vi "PockelsControl.vi"(8 "Error In":errorcluster, 10 "Laser Power (%)":dbl max=100.0 step=1.0) -> (0 "Error Out":errorcluster)   [LabVIEW 2013]
uses:
  Peripherals Control/Shutter/Typedefs/Shutter state.ctl
  Typedefs/HW config states enum.ctl
  <vilib>/DAQmx/write.llb/DAQmx Write (Analog DBL 1Chan 1Samp).vi
  Global Variables/General Globals.vi
  Global Variables/gl_UI Ctrl Refs.vi
  Peripherals Control/Pockels/Globals/gl_Pockels control globals.vi
  <vilib>/DAQmx/create/channels.llb/DAQmx Create Channel (AO-Voltage-Basic).vi
  <vilib>/DAQmx/miscellaneous.llb/DAQmx Fill In Error Info.vi
panel:
  out "DAQmx Physical Channel":tag="PXI1Slot4/ao0"
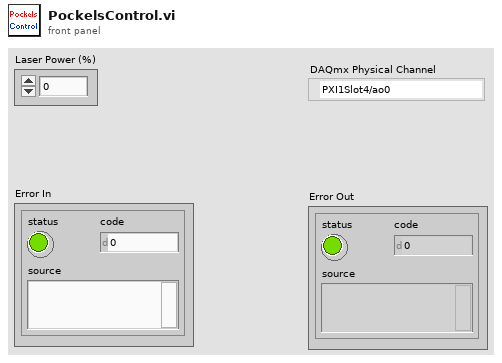
[diagram p1: front panel]
types:
  T1 = typedef "Shutter state.ctl" = enum16{"Closed/Disabled", "Open/Enabled"}
  T2 = typedef "HW config states enum.ctl" = enum16{"Load from file", "Save to file", "Write all", "Read all", "Write XY stage settings", "Write DAQ FPGA settings", "Write Control FPGA settings", "Write Phys Channels", "Clear", "Compare from file"}
  T3 = typedef "Sys Configuration.ctl" = cluster{"XY Stage":T4, "DAQ FPGA":T5, "Control system":T9, "Encoder":T10, "DAQmx Chan":T11, "Computer MAC address":string, "Cam VidRec":T12, "Externalise Triggers":bool, "Laser wavelength (nm)":dbl}
  T4 = typedef "XY Stage config cluster.ctl" = cluster{"COM port":refnum<visa-resource-name>, "XY stage available":bool}
  T5 = typedef "DAQ FPGA config cluster.ctl" = cluster{"Ref":T6, "Target":T7, "Clock Freq (MHz) ":dbl, "input card type":T8, "Samples Wait after Trigger":u16, "AOD fill":u16, "StartupDelay":i32, "Slip Cycle (clock cycles)":u32, "Add Cycle":bool}
  T6 = typedef "FPGA Ref.ctl" = refnum<k20>
  T7 = typedef "nirio_resource_hc.ctl" = tag
  T8 = typedef "FPGA input type AC-DC.ctl" = enum16{"AC Card", "DC Card"}
  T9 = typedef "CTRL system config cluster.ctl" = cluster{"Ethernet opened":bool, "Ethernet Port":u32, "Ctrl FPGA available":bool, "Ctrl FPGA Clock (MHz)":dbl, "Ctrl system MAC address":string, "Control system.Network adapter name":string, "AOD 1 Amplitude":i16, "AOD 2 Amplitude":i16, "AOD 3 Amplitude":i16, "AOD 4 Amplitude":i16, "Data Time Interval (ns)":dbl, "T0 (ns)":dbl, "Ta (ns)":dbl}
  T10 = typedef "Encoder config cluster.ctl" = cluster{"IP address":string, "Port":u16, "Encoder available":bool, "Wheel radius (cm)":dbl}
  T11 = typedef "DAQmx physical channels cluster.ctl" = cluster{"Pockels AO":tag, "Hard shutter AO":tag, "PMT AOs":tag, "Power meter AI":tag}
  T12 = typedef "Cam VidRec HW config setup cluster.ctl" = cluster{"DO flag-Video record":tag, "DO flag-Trial start":tag, "VidRec available":bool}
  T13 = typedef "UI ctrl refs cluster.ctl" = cluster{"Top level VI path":path, "Top level VI ref":refnum<vi>, "User menu ref":refnum<k9>, "Sub Panel control":refnum<vi>, "Imaging Param Tab":refnum<vi>, "Occurrence-Start drivers":refnum<k4>, "Occurrence-Speed logging initialised":refnum<k4>, "Occurrence-XYZ stage initialised":refnum<k4>, "Exit button":refnum<vi>, "Status ind":refnum<vi>, "Return to Origin":refnum<vi>, "Speed Logging":refnum<vi>, "Time Lapse":refnum<vi>, "Live Imaging":refnum<vi>, "AOL Z Stack":refnum<vi>, "Motor Z Stack":refnum<vi>, "Funct Acq button":refnum<vi>, "Hard Shutter":refnum<vi>, "Virtual Shutter":refnum<vi>, "Laser Power":refnum<vi>, "AOL Mode":refnum<vi>, "Frame Size":refnum<vi>, "Field of View":refnum<vi>, "Dwell Time":refnum<vi>, "Zoom":refnum<vi>, "AOL Z":refnum<vi>, "Objective":refnum<vi>, "Axis":refnum<vi>, "Paths & Names":refnum<vi>, "Experiment folder path (ind.)":refnum<vi>, "Last State (Ind.)":refnum<vi>, "Laser wavelength ind (nm)":refnum<vi>, "Averages":refnum<vi>, "Angle (degrees)":refnum<vi>, "X centre":refnum<vi>, "Y centre":refnum<vi>, "Plane Mode":refnum<vi>, "# Planes":refnum<vi>, "Z Start":refnum<vi>, "Z Stop":refnum<vi>, "Z Step":refnum<vi>, "PMT 1":refnum<vi>, "PMT 2":refnum<vi>, "Stage XYZ Position":refnum<vi>, "Pockels@Z Start":refnum<vi>, "Pockels@Z Stop":refnum<vi>, "Obtain Z Start":refnum<vi>, "Obtain Z Stop":refnum<vi>, "Live stim.trig.period":refnum<vi>, "Live stim.trig.enable":refnum<vi>, "Funct. Acq. Pockels Modulation":refnum<vi>, "Enable Video Recording":refnum<vi>, "Video Record-Live Imaging":refnum<vi>, "Video Record-Funct acq":refnum<vi>, "AOL Z-stack Chirps Ready (ind)":refnum<vi>, "Center freq ind (nm)":refnum<vi>, "Logging queue (ind)":refnum<vi>, "Back aperture power (ind.)":refnum<vi>, "Power after objective (ind.)":refnum<vi>, "Switch user":refnum<vi>}
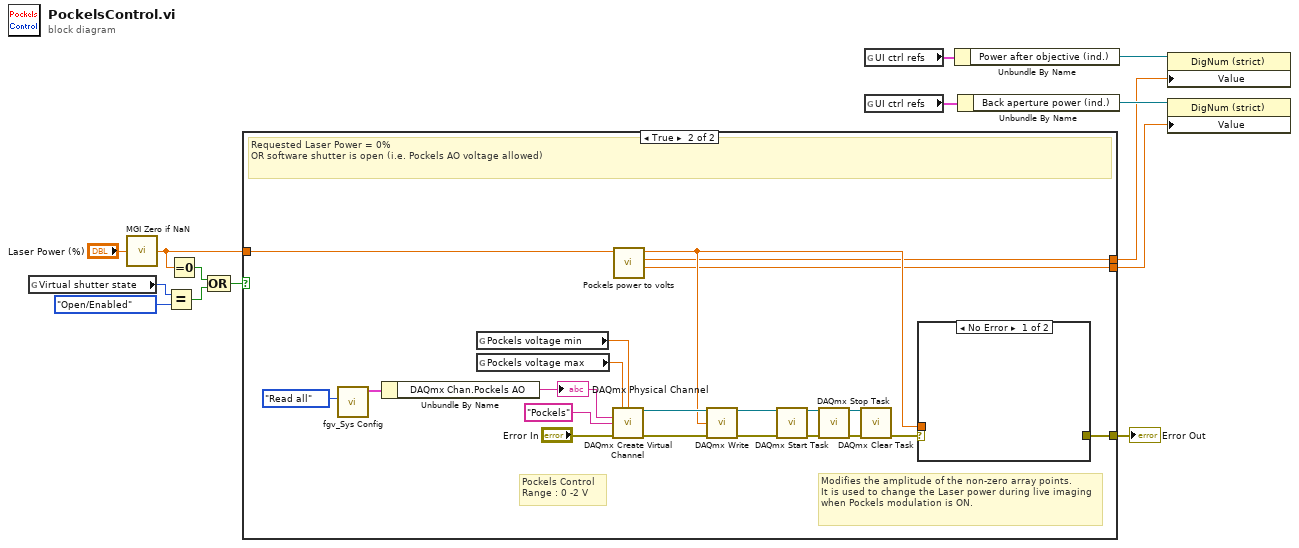
[diagram p0: block diagram]
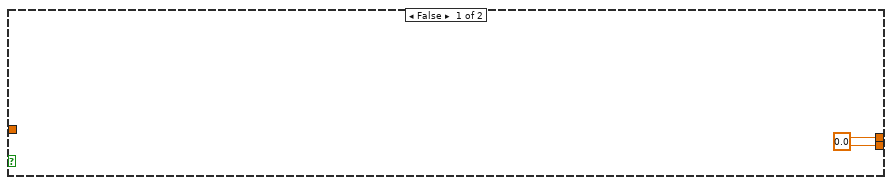
[diagram p2: hidden frame]
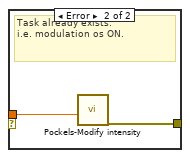
[diagram p3: hidden frame]
diagram:
  n1 = global read "General Globals.vi" "Virtual shutter state"() -> (w10:T1)
  n2 = call <userlib>:"MGI Zero if NaN.vi"("Number In"="Laser Power (%)") -> ("Number Out"=w1:dbl)
  n3 = Equal?(x=w10, y=Shutter_state."Open/Enabled") -> (x = y?=w11:bool)
  n4 = Equal To 0?(x=w1) -> (x = 0?=w12:bool)
  n5 = Compound Arithmetic op=OR(w12, w11) -> (w9:bool)
  n6 = case shown="True" w9 {
    tunnel: [_ w26] -> w14
    tunnel: w1 -> [_ w24]
    tunnel: [w15 w17] -> w6
    tunnel: [w15 w16] -> w3
    frame False {
      w15 = 0.0 ("Normalised power (mW)")
    }
    frame True {
      # "Modifies the amplitude of the non-zero array points.\nIt is used to change the Laser power during live imaging when Pockels modulation is ON."
      # "Pockels Control\nRange : 0 -2 V"
      # "Requested Laser Power = 0%\nOR software shutter is open (i.e. Pockels AO voltage allowed)"
      n7 = call "fgv_Sys Config.vi"("Function"=HW_config_states_enum."Read all") -> ("System Config out"=w19:T3)  [unwired: 9 in, 1 out]
      n8 = Unbundle By Name(w19) -> ("DAQmx Chan.Pockels AO"=w18:tag)
      "DAQmx Physical Channel" <- w18
      n9 = global read "gl_Pockels control globals.vi" "Pockels voltage min"() -> (w23:dbl)
      n10 = global read "gl_Pockels control globals.vi" "Pockels voltage max"() -> (w22:dbl)
      n11 = call-poly <vilib>:"DAQmx Create Virtual Channel.vi"("maximum value"=w22, "minimum value"=w23, "physical channels"=w18, "name to assign"="Pockels", "error in"="Error In") -> ("task out"=w36:refnum<k21>, "error out"=w35:errorcluster)  [unwired: 9 in]
      n12 = call "Pockels power to volts.vi"("Pockels power (%)"=w24) -> ("Back-aperture power (mW)"=w17:dbl, "Power after the objective (mW)"=w16:dbl, "Pockels control voltage (V)"=w21:dbl)  [unwired: 8 in]
      n13 = call-poly <vilib>:"DAQmx Write.vi"("task/channels in"=w36, "data"=w21, "error in"=w35) -> ("task out"=w34:refnum<k21>, "error out"=w33:errorcluster)  [unwired: 10 in, 1 out]
      n14 = call <vilib>:"DAQmx Start Task.vi"("task/channels in"=w34, "error in"=w33) -> ("task out"=w27:refnum<k21>, "error out"=w28:errorcluster)  [unwired: 12 in]
      n15 = call <vilib>:"DAQmx Stop Task.vi"("task/channels in"=w27, "error in"=w28) -> ("task out"=w32:refnum<k21>, "error out"=w31:errorcluster)  [unwired: 12 in]
      n16 = call <vilib>:"DAQmx Clear Task.vi"("task in"=w32, "error in"=w31) -> ("error out"=w25:errorcluster)  [unwired: 13 in]
      n17 = case shown="No Error" w25 {
        tunnel: [_ w38] -> w26
        tunnel: w21 -> [_ w37]
        frame No Error {
        }
        frame Error {
          # "Task already exists.\ni.e. modulation os ON."
          n18 = call "Pockels-Modify intensity.vi"("Pockels control value (V)"=w37) -> ("error out"=w38:errorcluster)  [unwired: 9 in, 1 out]
        }
      }
    }
  }
  "Error Out" <- w14
  n19 = global read "gl_UI Ctrl Refs.vi" "UI ctrl refs"() -> (w4:T13)
  n20 = global read "gl_UI Ctrl Refs.vi" "UI ctrl refs"() -> (w8:T13)
  n21 = Unbundle By Name(w4) -> ("Power after objective (ind.)"=w5:refnum<vi>)
  n22 = Unbundle By Name(w8) -> ("Back aperture power (ind.)"=w7:refnum<vi>)
  n23 = property class="DigNum (strict)"(reference=w5, "Value"=w3) -> ()  [unwired: 1 in, 2 out]
  n24 = property class="DigNum (strict)"(reference=w7, "Value"=w6) -> ()  [unwired: 1 in, 2 out]
